vi "Ellipiticity.vi"(2 "S or L":dbl, 3 "P or R":dbl) -> (0 "P+S":dbl, 1 "(P-S)/(P+S)":dbl)   [LabVIEW 2020, in "SignalConverson.lvlib"]
uses:
  SignalConverson.lvlib
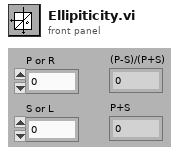
[diagram p1: front panel]
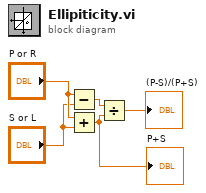
[diagram p0: block diagram]
diagram:
  n1 = Subtract(x="P or R", y="S or L") -> (x-y=w2:dbl)
  n2 = Add(x="P or R", y="S or L") -> (x+y=w1:dbl)
  "P+S" <- w1
  n3 = Divide(x=w2, y=w1) -> (x/y=→"(P-S)/(P+S)":dbl)
